vi "get desired keys.vi"(8 "error in":errorcluster, 11 "fixed channel tag bus module configuration in":refnum<class "user control module configuration.lvclass">) -> (0 "error out":errorcluster, 2 "desired keys":string[](array[string]), 3 "fixed channel tag bus module configuration out":refnum<class "user control module configuration.lvclass">)   [LabVIEW 2013, in "user control module configuration.lvclass"]
uses:
  user control module configuration.lvclass
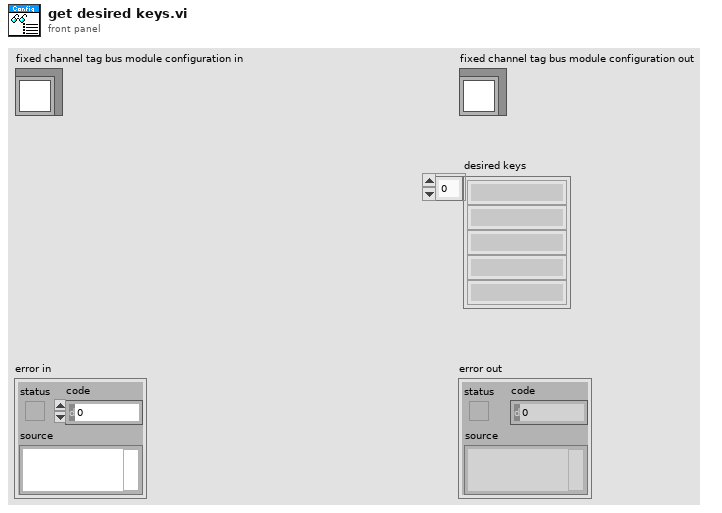
[diagram p1: front panel]
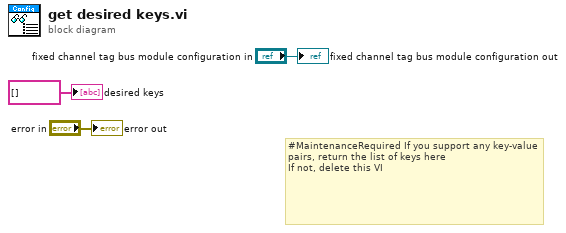
[diagram p0: block diagram]
diagram:
  # "#MaintenanceRequired If you support any key-value pairs, return the list of keys here\nIf not, delete this VI"
  "error out" <- "error in"
  "fixed channel tag bus module configuration out" <- "fixed channel tag bus module configuration in"
  "desired keys" <- string[] [] ("desired keys")
